vi "LINX - Blink + Measure -- SwitchError.vi"() -> ()   [LabVIEW 2025]
doc: "Automatically blink and LED attached to a digital output channel of a LINX device."
uses:
  <vilib>/MakerHub/LINX/Public/Peripherals/Digital/Digital Write 1 Chan.vi
  <vilib>/MakerHub/LINX/Public/Peripherals/Analog/Analog Read 1 Chan.vi
  <vilib>/MakerHub/LINX/Public/Peripherals/Digital/Digital Write N Chans.vi
  <vilib>/MakerHub/LINX/Public/Peripherals/Analog/Analog Read N Chans.vi
  <vilib>/MakerHub/LINX/Private/Local IO/LinxDigitalWrite.vi
  <vilib>/MakerHub/LINX/Public/Utilities/Check Channel.vi
  <vilib>/MakerHub/LINX/Private/Local IO/LinxAnalogRead.vi
  <vilib>/MakerHub/LINX/Public/Utilities/Open Serial.vi
  <vilib>/MakerHub/LINX/Private/Utilties/Generate Error.vi
  <vilib>/MakerHub/LINX/LMH-LINX.lvlib
panel:
  in  "MeasStop Button":bool
  in  "AI Channel":u8
  out "Meas Loop Rate (Hz)":u32
  out "Analog Data":dbl(graph)
  in  "WaitTime (sec)":dbl(slide) scale=0.01..1.0
  out "LED Value":bool
  in  "Digital Output Channel":u8=13
  in  "Serial Port":refnum<visa-resource-name>
  out "Src Loop Rate (Hz)":u32
  in  "Stop Button":bool
  # "Circuit Schematic"
  # "LINX Device Settings"
  # "LED Value"
  # "Blink (Serial Interface)\n\nThis example demonstrates how to blink an LED on a LINX device connected to \nthe host computer using USB / Serial.\n\nInstructions\n1. Select the Serial Port associated with the LINX Device.\n2. Select the Digital Pin connected to the LED.\n3. Click the Run Arrow."
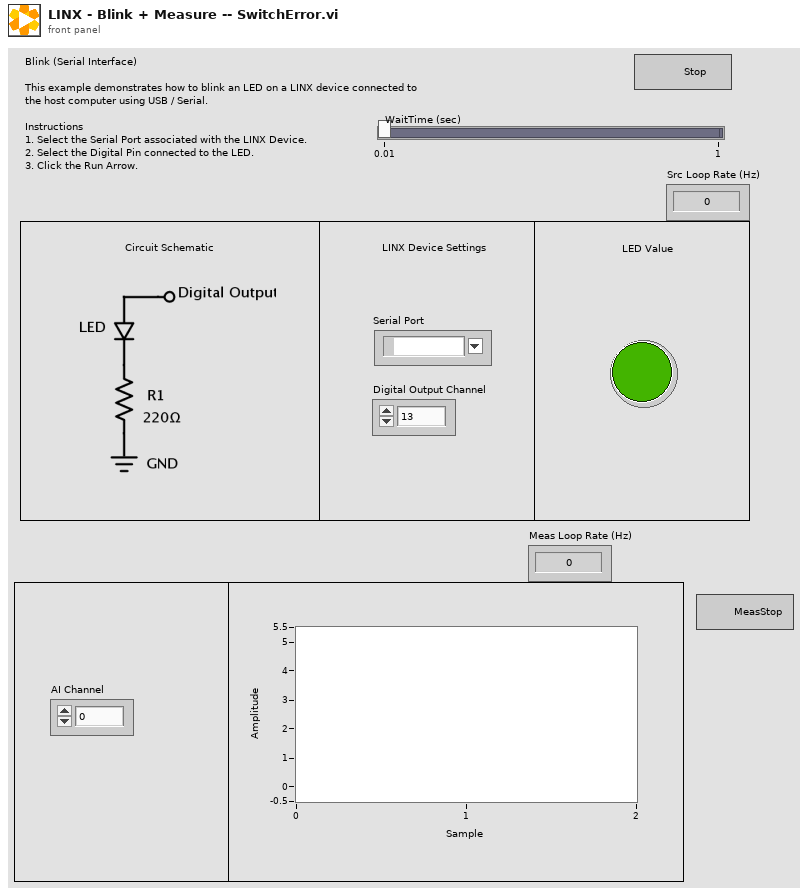
[diagram p1: front panel]
types:
  T1 = typedef "LMH-LINX.lvlib/LINX Ref.ctl" = cluster{"IO":T2, "Interface":T3, "LINX Device Config":T4}
  T2 = typedef "LMH-LINX.lvlib/Platform.ctl" = enum16{"Remote", "Local"}
  T3 = typedef "LMH-LINX.lvlib/Interface.ctl" = enum16{"Serial", "TCP"}
  T4 = typedef "LMH-LINX.lvlib/Device.lvlib/LINX Device Config.ctl" = cluster{"Interface":T3, "COM Port":refnum<visa-resource-name>, "TCP Configuration":T5, "Device Family":u8, "Device ID":u8, "Device Name":string, "TCP Ref":refnum<k5>, "Channels":T6}
  T5 = typedef "LMH-LINX.lvlib/Device.lvlib/TCP Config.ctl" = cluster{"IP Address":string, "Port":u16}
  T6 = typedef "LMH-LINX.lvlib/Channels.ctl" = cluster{"DI":u8[], "DO":u8[], "AI":u8[], "AO":u8[], "PWM":u8[], "QE":u8[], "UART":u8[], "I2C 2":u8[], "SPI":u8[], "CAN":u8[], "Servo":u8[], "AI Ref (V)":dbl, "AI Resolution (Bits)":u8, "AO Ref (V)":dbl, "AO Resolution (Bits)":u8}
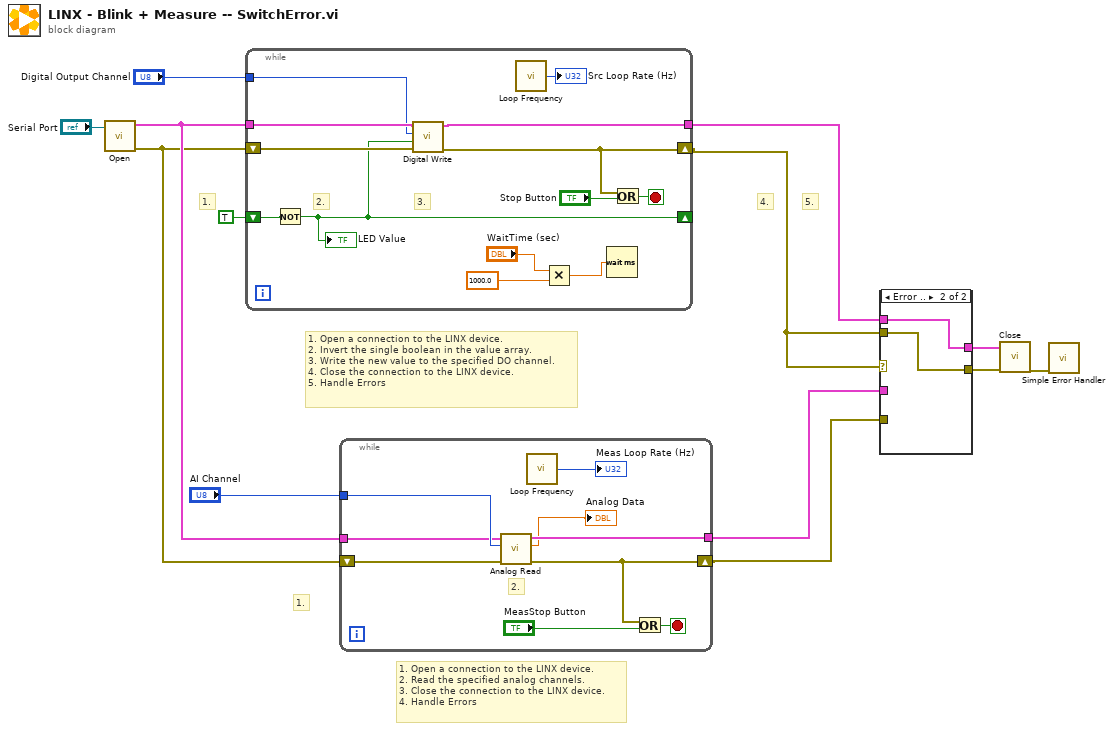
[diagram p0: block diagram]
diagram:
  # "1. Open a connection to the LINX device.\n2. Read the specified analog channels.\n3. Close the connection to the LINX device.\n4. Handle Errors"
  # "1."
  # "1. Open a connection to the LINX device.\n2. Invert the single boolean in the value array.\n3. Write the new value to the specified DO channel.\n4. Close the connection to the LINX device.\n5. Handle Errors"
  # "5."
  # "4."
  # "1."
  n1 = call-poly <vilib>:"Open.vi"("Serial Port"="Serial Port") -> ("Error Out"=w7:errorcluster, "LINX Resource"=w8:T1)  [unwired: 8 in, 1 out]
  n2 = while {
    tunnel: w8 -> [w24]
    tunnel: [w23] -> w5
    shift-right: [w21] -> w3
    shift-left: w7 -> [w22]
    shift-right: [w18] -> _
    shift-left: TRUE -> [w19]
    tunnel: "Digital Output Channel" -> [w20]
    stop <- w26 stop-if-true
    # "2."
    # "3."
    n3 = Not(x=w19) -> (.not. x?=w18:bool)
    "LED Value" <- w18
    n4 = call-poly <vilib>:"Digital Write.vi"("Error In"=w22, "Output Value"=w18, "DO Channel"=w20, "LINX Resource"=w24) -> ("Error Out"=w21:errorcluster, "LINX Resource"=w23:T1)  [unwired: 6 in]
    n5 = call <vilib>:"Loop Frequency.vi"() -> ("Loop Rate (Hz)"=→"Src Loop Rate (Hz)":u32)
    n6 = Multiply(x="WaitTime (sec)", y=1000.0) -> (x*y=w17:dbl)
    n7 = Wait (ms)(milliseconds to wait=w17) -> ()  [unwired: 1 out]
    n8 = Or(x=w21, y="Stop Button") -> (x .or. y?=w26:bool)
  }
  n9 = while {
    tunnel: [w34] -> w1
    shift-right: [w32] -> w2
    shift-left: w7 -> [w35]
    tunnel: "AI Channel" -> [w31]
    tunnel: w8 -> [w28]
    stop <- w33 stop-if-true
    # "2."
    n10 = call-poly <vilib>:"Analog Read.vi"("Error In"=w35, "Analog Channel"=w31, "LINX Resource"=w28) -> ("Error Out"=w32:errorcluster, "Voltage"=→"Analog Data":dbl, "LINX Resource"=w34:T1)  [unwired: 5 in, 1 out]
    n11 = call <vilib>:"Loop Frequency.vi"() -> ("Loop Rate (Hz)"=→"Meas Loop Rate (Hz)":u32)
    n12 = Or(x=w32, y="MeasStop Button") -> (x .or. y?=w33:bool)
  }
  n13 = case shown="Error .." w3 {
    tunnel: [w36 w39] -> w6
    tunnel: w5 -> [_ w39]
    tunnel: [w37 w38] -> w4
    tunnel: w3 -> [_ w38]
    tunnel: w2 -> [w37 _]
    tunnel: w1 -> [w36 _]
    frame No Error {
    }
    frame Error {
    }
  }
  n14 = call <vilib>:"Close.vi"("Error In"=w4, "LINX Resource"=w6) -> ("Error Out"=w13:errorcluster)  [unwired: 9 in]
  n15 = call <vilib>:"Simple Error Handler.vi"("error in (no error)"=w13) -> ()  [unwired: 4 in, 5 out]
